vi "信息框（标题、文本、图标）.vi"(7 "icon":i32(ring) items=["None"=0, "Hand, Error, Stop"=16, "Question"=32, "Exclamation, Warning"=48, "Asterisk, Information"=64], 8 "错误输入（无错误）":errorcluster, 9 "buttons":i32(ring) items=["OK", "OKCancel", "AbortRetryIgnore", "YesNoCancel", "YesNo", "RetryCancel"], 10 "caption":string, 11 "text":string) -> (0 "错误输出":errorcluster, 3 "按钮输出":i32(ring) items=["None", "OK", "Cancel", "Abort", "Retry", "Ignore", "Yes", "No"])   [LabVIEW 2020]
uses:
  System.Windows.Forms
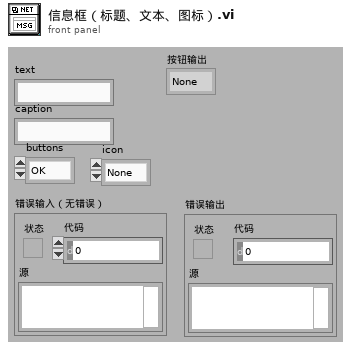
[diagram p1: front panel]
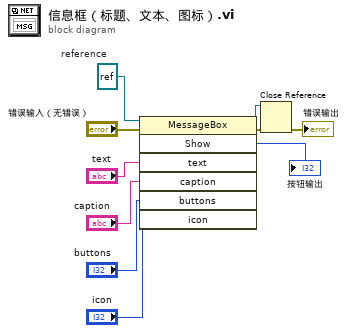
[diagram p0: block diagram]
diagram:
  w5 = refnum<k24> refnum  # reference
  n1 = invoke class="MessageBox" method="Show"(reference=w5, error in="错误输入（无错误）", "text"="text", "caption"="caption", "buttons"="buttons", "icon"="icon") -> (reference out=w10:refnum<k24>, error out=w9:errorcluster, "Show"=→"按钮输出":i32)  [unwired: 1 in, 4 out]
  n2 = Close Reference(reference=w10, error in (no error)=w9) -> (error out=→"错误输出":errorcluster)
